vi "Shooter Controller.vi"(8 "error in":errorcluster) -> ()   [LabVIEW 2020]
doc: "This VI executes continuously carrying out the current operation and responding to updates or new operations. It will often contain the timing or control code that is difficult to place directly in TeleOp. This VI generally opens all sensors and motors and isolates the rest of the robot code from knowing how the operations are carried out."
uses:
  <vilib>/Rock Robotics/WPI/Framework/Completion Status.ctl
  Shooter Setpoints.ctl
  Shooter Operations.ctl
  <vilib>/Rock Robotics/WPI/SafetyOutput/WPI_SafetyOutputConfigMenu.ctl
  <vilib>/Rock Robotics/Network Tables/NT Write Number.vi
panel:
  in  "Interactive Values":T1
  out "Current\nCmd":string
  in  "Buttons":cluster{"Execute Cmd":bool, "Abort Cmd":bool}
  out "Command Timing":cluster{"Start Time (ms)":u32, "Iterations":i32}
  out "Status":T3
  # "Tip: It may be helpful to observe inputs and sensor values.\nYou may also want to display tuning or debugging controls."
  # "Interactive Command: You may fill in the settings for a command\nand schedule it with the Execute button. You can observe and abort\nany command while fine tuning the code for the controller."
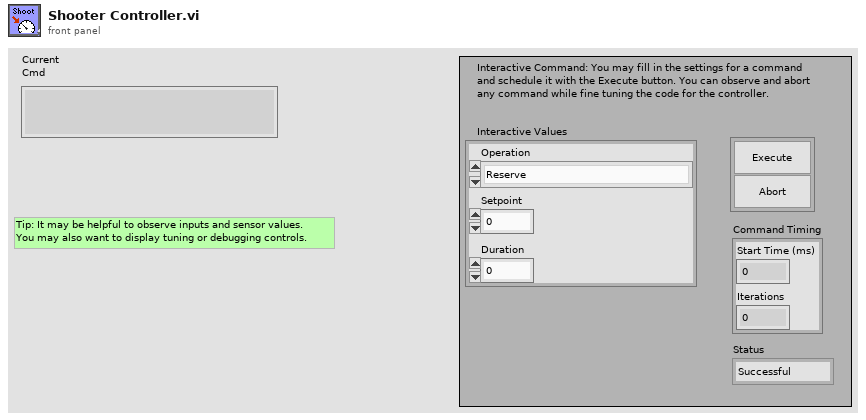
[diagram p1: front panel]
types:
  T1 = typedef "Shooter Setpoints.ctl" = cluster{"Operation":T2, "Setpoint":dbl, "Duration":dbl}
  T2 = typedef "Shooter Operations.ctl" = enum16{"Reserve", "Read Current", "Immediate", "for Time"}
  T3 = typedef "Completion Status.ctl" = enum16{"Successful", "Aborted", "Incomplete"}
  T4 = typedef "WPI_SafetyOutputConfigMenu.ctl" = enum16{"Enable", "Disable"}
  T5 = typedef "WPI_MotorControlDeviceRef.ctl" = cluster{"DeviceStatus":errorcluster, "Type":T6, "PWM":cluster{"PWM Channel":T7, "DeadBand":T8}, "CAN":cluster{"Device Number":u8, "SetOutput VI Ref":variant, "GetOutput VI Ref":variant, "Enable VI Ref":variant, "Disable VI Ref":variant, "Data":variant}, "Invert":bool, "DIO PWM":cluster{"PWM \"Enable\" Channel":T7, "DIOChannel":T9, "PWM Rate":dbl}}
  T6 = typedef "WPI_MotorControlType.ctl" = enum16{"PWM", "CAN", "DIO PWM"}
  T7 = typedef "FPGA_DIOPWMChannel.ctl" = enum8{"PWM 0", "PWM 1", "PWM 2", "PWM 3", "PWM 4", "PWM 5", "PWM 6", "PWM 7", "PWM 8", "PWM 9", "PWM MXP 0", "PWM MXP 1", "PWM MXP 2", "PWM MXP 3", "PWM MXP 4", "PWM MXP 5", "PWM MXP 6", "PWM MXP 7", "PWM MXP 8", "PWM MXP 9", "Invalid"}
  T8 = typedef "WPI_PWMDeadband.ctl" = cluster{"Name":string, "maxPositivePwm":i32, "minPositivePwm":i32, "centerPwm":i32, "maxNegativePwm":i32, "minNegativePwm":i32, "angularRange":u16}
  T9 = typedef "FPGA_DIOChannel.ctl" = enum8{"DIO 0", "DIO 1", "DIO 2", "DIO 3", "DIO 4", "DIO 5", "DIO 6", "DIO 7", "DIO 8", "DIO 9", "DIO MXP 0", "DIO MXP 1", "DIO MXP 2", "DIO MXP 3", "DIO MXP 4", "DIO MXP 5", "DIO MXP 6", "DIO MXP 7", "DIO MXP 8", "DIO MXP 9", "DIO MXP 10", "DIO MXP 11", "DIO MXP 12", "DIO MXP 13", "DIO MXP 14", "DIO MXP 15", "SPI Port CS1", "SPI Port CS2", "SPI Port CS3", "SPI Port MISO", "SPI Port MOSI", "Invalid"}
  T10 = typedef "Command Status Info.ctl" = cluster{"Name":string, "Status":T3, "notifier out":T11}
  T11 = typedef "Completion Notifier.ctl" = refnum<notifier>
  T12 = cluster{"Current Command":T1, "Command Timing":cluster{"Start Time (ms)":u32, "Iterations":i32}, "Command Arguments":cluster{"Command Info":T10, "Description":string, "Default Command":T1, "queue out":refnum<queue>, "Subsystem Name":string}}
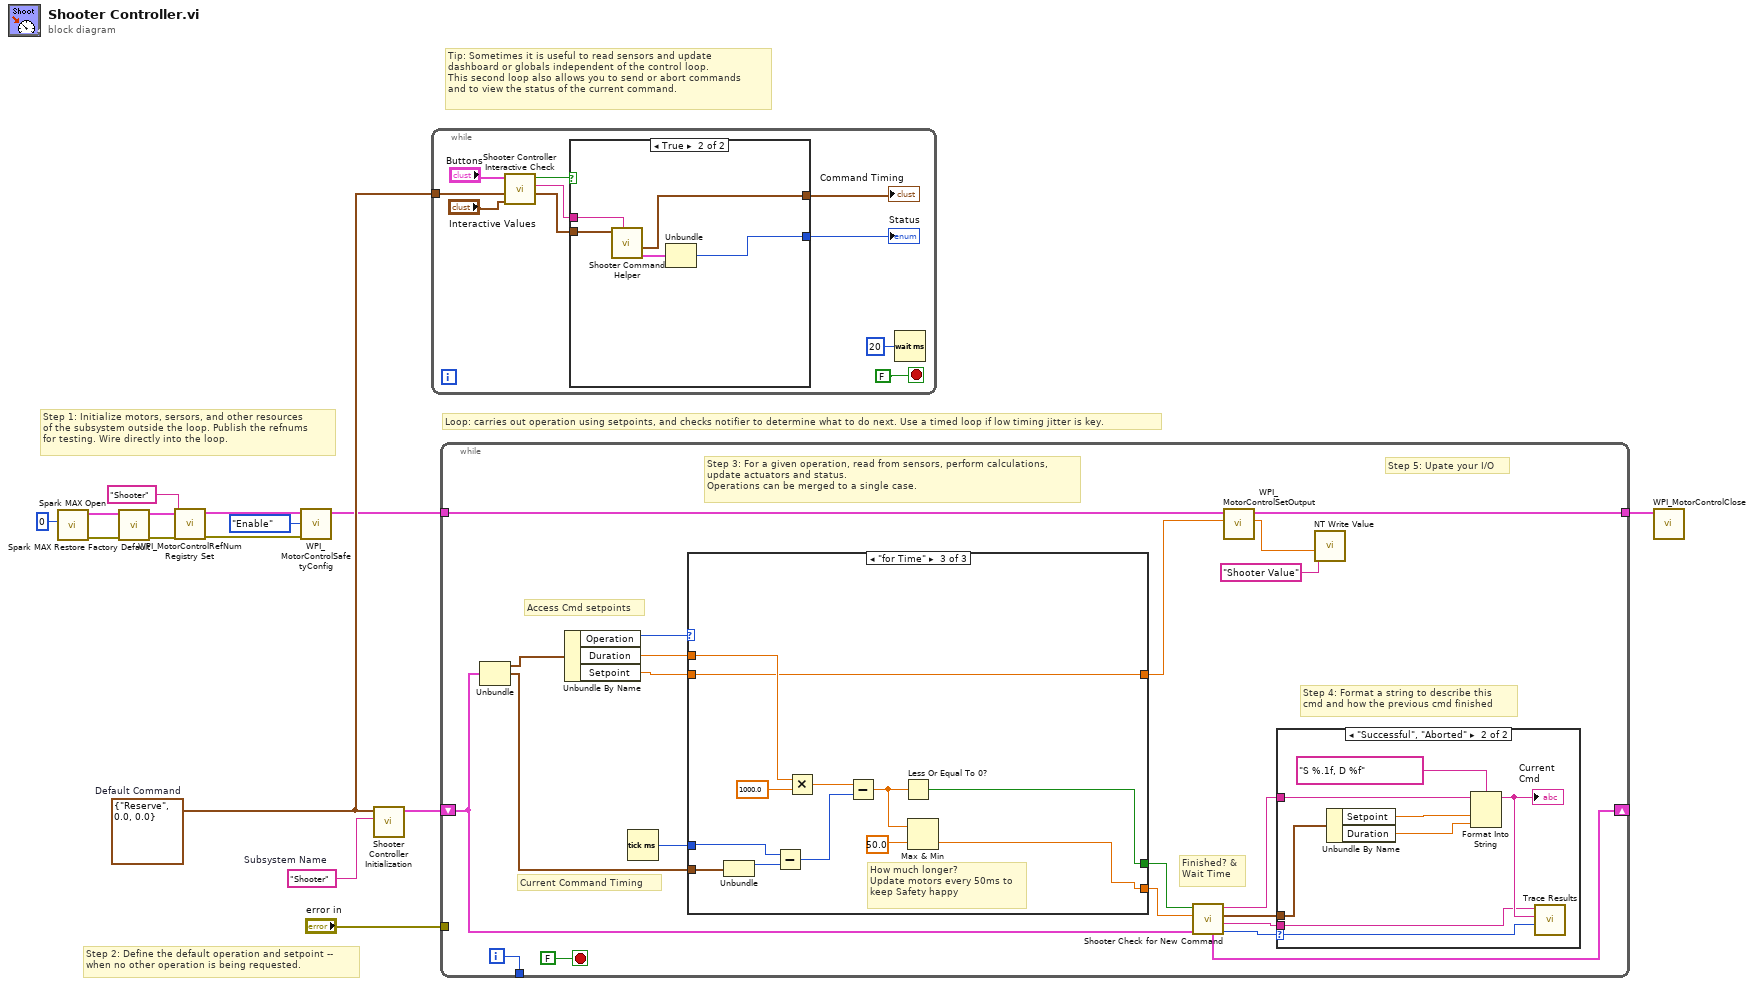
[diagram p0: block diagram]
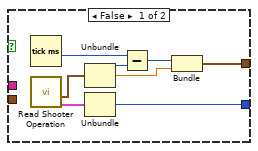
[diagram p2: hidden frame]
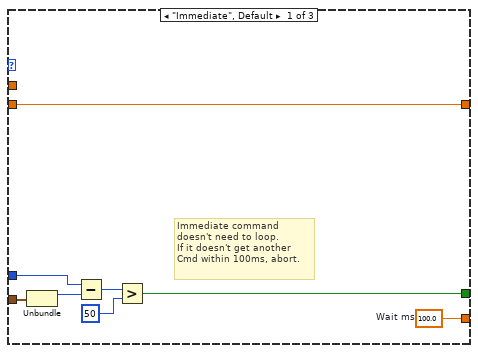
[diagram p4: hidden frame]
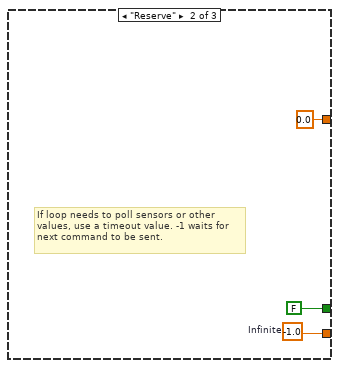
[diagram p5: hidden frame]
diagram:
  w12 = T1 {"Operation"=enum."Reserve", "Setpoint"=0.0, "Duration"=0.0}  # Default Command
  w13 = "Shooter"  # Subsystem Name
  # "Tip: Sometimes it is useful to read sensors and update\ndashboard or globals independent of the control loop.\nThis second loop also allows you to send or abort commands\nand to view the status of the current command."
  # "Step 2: Define the default operation and setpoint --\nwhen no other operation is being requested."
  # "Step 1: Initialize motors, sersors, and other resources\nof the subsystem outside the loop. Publish the refnums\nfor testing. Wire directly into the loop."
  # "Loop: carries out operation using setpoints, and checks notifier to determine what to do next. Use a timed loop if low timing jitter is key."
  n1 = call <vilib>:"Spark MAX Open.vi"("Device Number"=u8 0) -> ("error out"=w10:errorcluster, "MotorControlDeviceRef"=w9:T5)  [unwired: 9 in]
  n2 = call <vilib>:"Spark MAX Restore Factory Default.vi"("error in"=w10, "MotorControlDeviceRef"=w9) -> ("error out"=w7:errorcluster, "MotorControlDeviceRef"=w8:T5)  [unwired: 8 in]
  n3 = call <vilib>:"WPI_MotorControlRefNum Registry Set.vi"("error in (no error)"=w7, "refnum name"="Shooter", "MotorControlDevRef"=w8) -> ("error out"=w5:errorcluster, "MotorControlDevRef"=w4:T5)  [unwired: 7 in]
  n4 = call <vilib>:"WPI_MotorControlSafetyConfig.vi"("error in (no error)"=w5, "mode"=WPI_SafetyOutputConfigMenu."Enable", "MotorControlDevRef"=w4) -> ("MotorControlDevRef"=w2:T5)  [unwired: 7 in, 1 out]
  n5 = call "Shooter Controller Initialization.vi"("Subsystem Name"=w13, "Default Command"=w12) -> ("Current Command"=w14:T12)  [unwired: 9 in]
  n6 = while {
    tunnel: w12 -> [w22]
    stop <- FALSE stop-if-true
    n7 = call "Shooter Controller Interactive Check.vi"("Interactive Command in"="Interactive Values", "Default Command"=w22, "Buttons"="Buttons") -> ("Interactive Command out"=w19:T1, "Trace String"=w20:string, "Schedule"=w21:bool)  [unwired: 6 in]
    n8 = case shown="True" w21 {
      tunnel: [w33 w38] -> w18
      tunnel: w19 -> [_ w36]
      tunnel: [w29 w34] -> w17
      tunnel: w20 -> [_ w37]
      frame False {
        n9 = Tick Count (ms)() -> (millisecond timer value=w28:u32)
        n10 = call "Read Shooter Operation.vi"() -> ("Command Info"=w26:T10, "SubSystem Data"=w27:T1)  [unwired: 9 in, 1 out]
        n11 = Unbundle(w27) -> ("Operation"=w32:T2, "Setpoint"=w30:dbl)  [unwired: 1 out]
        n12 = Unbundle(w26) -> ("Status"=w33:T3)  [unwired: 2 out]
        n13 = Subtract(x=w28, y=w32) -> (x-y=w31:u32)
        n14 = Bundle(w31, "Setpoint"=w30) -> (w29:cluster{u32, "Setpoint":dbl})  [unwired: 1 in]
      }
      frame True {
        n15 = call "Shooter Command Helper.vi"("Description"=w37, "SubSystem Data"=w36) -> ("Command Info Out"=w35:T10, "Command Timing"=w34:cluster{"Start Time (ms)":u32, "Iterations":i32})  [unwired: 7 in, 1 out]
        n16 = Unbundle(w35) -> ("Status"=w38:T3)  [unwired: 2 out]
      }
    }
    "Status" <- w18
    "Command Timing" <- w17
    n17 = Wait (ms)(milliseconds to wait=u32 20) -> ()  [unwired: 1 out]
  }
  n18 = while {
    shift-right: [w51] -> _
    shift-left: w14 -> [w44]
    tunnel: [w58] -> _
    tunnel: "error in" -> [_]
    tunnel: w2 -> [w43]
    tunnel: [w42] -> w1
    i -> [w58]
    stop <- FALSE stop-if-true
    # "Step 5: Upate your I/O"
    # "Step 4: Format a string to describe this\ncmd and how the previous cmd finished"
    # "Current Command Timing"
    # "Access Cmd setpoints"
    # "Finished? &\nWait Time"
    # "Step 3: For a given operation, read from sensors, perform calculations,\nupdate actuators and status.\nOperations can be merged to a single case."
    n19 = Unbundle(w44) -> ("Current Command"=w57:T1, "Command Timing"=w53:cluster{"Start Time (ms)":u32, "Iterations":i32})  [unwired: 1 out]
    n20 = Unbundle By Name(w57) -> ("Operation"=w56:T2, "Duration"=w55:dbl, "Setpoint"=w52:dbl)
    n21 = Tick Count (ms)() -> (millisecond timer value=w54:u32)
    n22 = case shown="\"for Time\"" w56 {
      tunnel: [w75 w78 w81] -> w49
      tunnel: [w69 FALSE ("ignore previous (F)") w82] -> w50
      tunnel: w53 -> [w71 _ w83]
      tunnel: w55 -> [_ _ w80]
      tunnel: w54 -> [w70 _ w84]
      tunnel: w52 -> [w68 _ w79]
      tunnel: [w68 0.0 ("Setpoint") w79] -> w41
      frame "Immediate", Default {
        w75 = 100.0  # Wait ms
        # "Immediate command\ndoesn't need to loop.\nIf it doesn't get another\nCmd within 100ms, abort."
        n23 = Unbundle(w71) -> ("Start Time (ms)"=w74:u32)  [unwired: 1 out]
        n24 = Subtract(x=w70, y=w74) -> (x-y=w73:u32)
        n25 = Greater?(x=w73, y=u8 50 ("Left Motor")) -> (0:w69:bool)
      }
      frame "Reserve" {
        w78 = -1.0  # Infinite
        # "If loop needs to poll sensors or other\nvalues, use a timeout value. -1 waits for\nnext command to be sent."
      }
      frame "for Time" {
        # "How much longer?\nUpdate motors every 50ms to\nkeep Safety happy"
        n26 = Unbundle(w83) -> ("Start Time (ms)"=w87:u32)  [unwired: 1 out]
        n27 = Subtract(x=w84, y=w87) -> (x-y=w90:u32)
        n28 = Multiply(x=w80, y=1000.0) -> (x*y=w89:dbl)
        n29 = Subtract(x=w89, y=w90) -> (x-y=w86:dbl)
        n30 = Less Or Equal To 0?(x=w86) -> (x <= 0?=w82:bool)
        n31 = Max & Min(x=w86, y=50.0) -> (min(x,y)=w81:dbl)  [unwired: 1 out]
      }
    }
    n32 = call "Shooter Check for New Command.vi"("Current Command"=w44, "Wait time (ms)"=w49, "Finished?"=w50) -> ("Completion"=w45:T3, "Subsystem Name"=w46:string, "Current Command"=w47:T1, "Initial Trace String"=w48:string, "NextCommand"=w51:T12)  [unwired: 4 in]
    n33 = call <vilib>:"WPI_MotorControlSetOutput.vi"("Output"=w41, "MotorControlDevRef"=w43) -> ("Motor Output"=w40:dbl, "MotorControlDevRef"=w42:T5)  [unwired: 7 in, 1 out]
    n34 = case shown="\"Successful\", \"Aborted\"" w45 {
      selector: w45 -> [_ w67]
      tunnel: w48 -> [_ w63]
      tunnel: w47 -> [_ w64]
      tunnel: w46 -> [_ w60]
      frame "Incomplete", Default {
        # "Continuing current command"
      }
      frame "Successful", "Aborted" {
        # "Report and setup for next command"
        n35 = Unbundle By Name(w64) -> ("Setpoint"=w66:dbl, "Duration"=w61:dbl)
        n36 = Format Into String(format string="S %.1f, D %f", initial string=w63, w66, w61) -> (resulting string=w62:string)  [unwired: 1 in, 1 out]
        "Current\nCmd" <- w62
        n37 = call <vilib>:"Trace Results.vi"("Status of previous command"=w67, "Description"=w62, "Subsystem"=w60) -> ()  [unwired: 9 in]
      }
    }
    n38 = call-poly <vilib>:"NT Write Value.vi"("Numeric"=w40, "Name"="Shooter Value") -> ()  [unwired: 9 in, 1 out]
  }
  n39 = call <vilib>:"WPI_MotorControlClose.vi"("MotorControlDevRef"=w1) -> ()  [unwired: 10 in, 1 out]
